vi "Configure.vi"(8 "error in (no error)":errorcluster, 11 "Insight in":refnum<class "Insight.lvclass">) -> (0 "error out":errorcluster, 3 "Insight out":refnum<class "Insight.lvclass">)   [LabVIEW 2014, in "Insight.lvclass"]
uses:
  Insight.lvclass
  Insight.lvclass/Insight.ctl
panel:
  out "Finished":bool
  out "Calibrating":bool
  in  "File Path Control":path=path "\\\\192.168.1.100\\data"
  in  "Aprox. Req. Sweep Rate (kHz)":dbl=50000.0
  in  "OK Button":bool
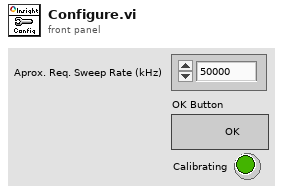
[diagram p1: front panel]
types:
  T1 = typedef "Telnet Session.ctl" = refnum<k1>
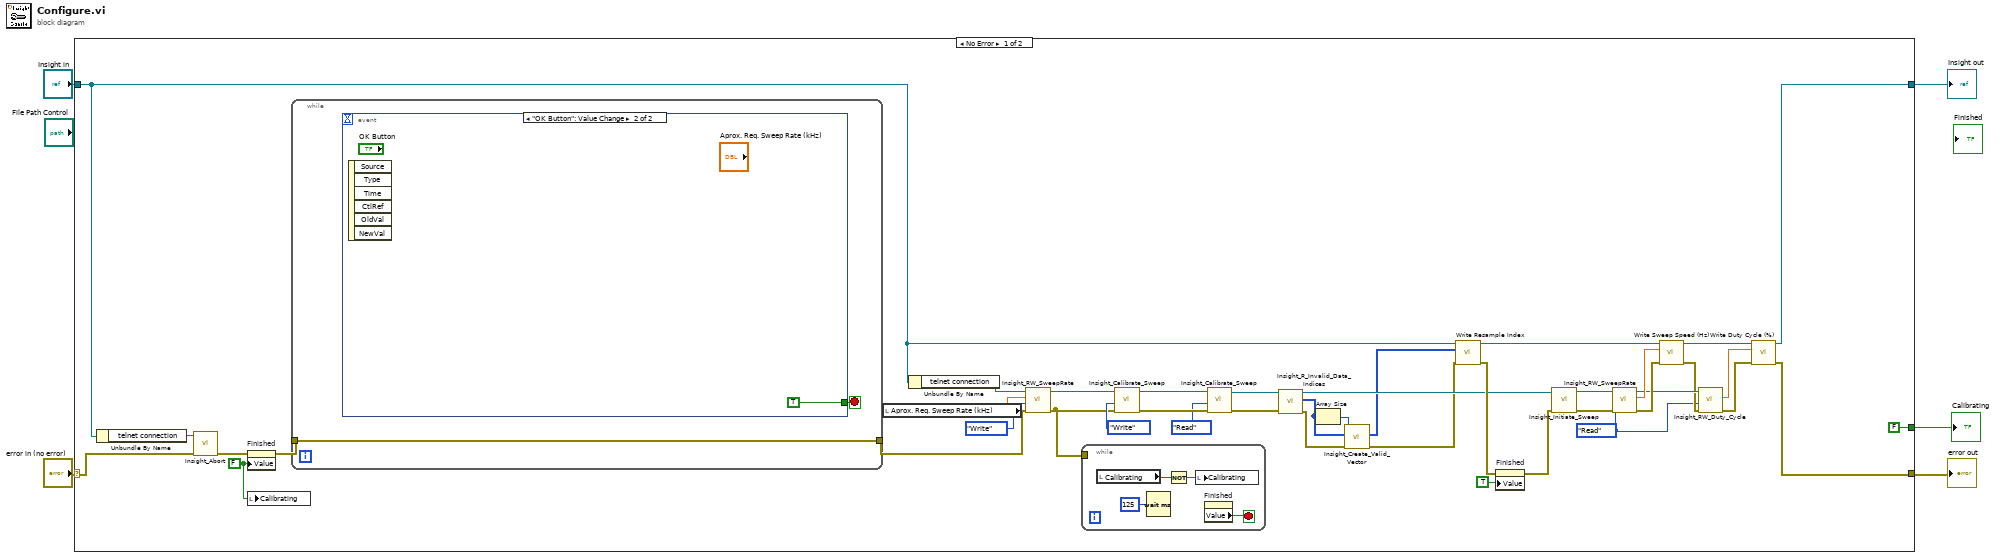
[diagram p0: block diagram]
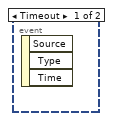
[diagram p2: hidden frame]
diagram:
  n1 = case shown="No Error" "error in (no error)" {
    selector: "error in (no error)" -> [w32 w56]
    tunnel: [w19 w56] -> w4
    tunnel: [w18 w55] -> w2
    tunnel: "Insight in" -> [w33 w55]
    tunnel: [FALSE _] -> w1
    frame No Error {
      w23 = enum8{"Write", "Read"}."Read" ("Mode (Read / Write)")
      w31 = FALSE ("Finished")
      n2 = Unbundle By Name(w33) -> ("telnet connection"=w34:T1)
      n3 = call "Insight_Abort.vi"("error in (no error)"=w32, "telnet connection"=w34) -> ("error out"=w35:errorcluster)  [unwired: 7 in, 2 out]
      n4 = property on="Finished" class="Bool (strict)"(error in=w35, "Value"=w31) -> (error out=w38:errorcluster)  [unwired: 1 in, 1 out]
      n5 = local write "Calibrating"(w31) -> ()
      n6 = while {
        tunnel: w38 -> [w52]
        tunnel: [w52] -> w41
        stop <- w53 stop-if-true
        n7 = event shown="[1] \"OK Button\": Value Change" {
          selector: _ -> [_ _]
          dyn-events: _ -> [_ _]
          timeout: _ -> [_ _]
          tunnel: [_ TRUE] -> w53
          event Timeout {
            n8 = event-data() -> ()  [unwired: 1 in, 3 out]
          }
          event "OK Button": Value Change {
            n9 = event-data() -> ()  [unwired: 1 in, 6 out]
          }
        }
      }
      n10 = local read "Aprox. Req. Sweep Rate (kHz)"() -> (w44:dbl)
      n11 = Unbundle By Name(w33) -> ("telnet connection"=w46:T1)
      n12 = call "Insight_RW_SweepRate.vi"("error in (no error)"=w41, "Mode (Read / Write)"=enum8{"Write", "Read"}."Write", "Sweep Rate (kHz)"=w44, "telnet connection"=w46) -> ("error out"=w40:errorcluster, "telnet  connection out"=w42:T1)  [unwired: 4 in, 2 out]
      n13 = while {
        tunnel: [w51] -> _
        tunnel: w40 -> [w51]
        stop <- w50 stop-if-true
        n14 = local read "Calibrating"() -> (w49:bool)
        n15 = Wait (ms)(milliseconds to wait=u32 125) -> ()  [unwired: 1 out]
        n16 = Not(x=w49) -> (.not. x?=w48:bool)
        n17 = local write "Calibrating"(w48) -> ()
        n18 = property on="Finished" class="Bool (strict)"() -> ("Value"=w50:bool)  [unwired: 2 in, 2 out]
      }
      n19 = call "Insight_Calibrate_Sweep.vi"("error in (no error)"=w40, "Mode (Read / Write)"=enum8{"Write", "Read"}."Write", "telnet connection"=w42) -> ("error out"=w16:errorcluster, "telnet  connection out"=w15:T1)  [unwired: 6 in, 1 out]
      n20 = call "Insight_Calibrate_Sweep.vi"("error in (no error)"=w16, "Mode (Read / Write)"=enum8{"Write", "Read"}."Read", "telnet connection"=w15) -> ("error out"=w10:errorcluster, "telnet  connection out"=w9:T1)  [unwired: 6 in, 1 out]
      n21 = call "Insight_R_Invalid_Data_Indices.vi"("error in (no error)"=w10, "telnet connection"=w9) -> ("error out"=w13:errorcluster, "Invalid Data Indices"=w11:i32[], "telnet  connection out"=w8:T1)  [unwired: 6 in, 1 out]
      n22 = Array Size(array=w11) -> (size(s)=w12:i32)
      n23 = call "Insight_Create_Valid_Vector.vi"("error in (no error)"=w13, "Invalid Data Indices"=w11, "total data length"=w12) -> ("error out"=w7:errorcluster, "Valid Vector"=w6:i32[])  [unwired: 7 in]
      n24 = call-dynamic "Write Resample Index.vi"("error in (no error)"=w7, "Resample Index"=w6, "Laser in"=w33) -> ("error out"=w37:errorcluster, "Laser out"=w26:refnum<class "Insight.lvclass">)  [unwired: 7 in]
      n25 = property on="Finished" class="Bool (strict)"(error in=w37, "Value"=TRUE ("Finished")) -> (error out=w36:errorcluster)  [unwired: 1 in, 1 out]
      n26 = call "Insight_Initiate_Sweep.vi"("error in (no error)"=w36, "telnet connection"=w8) -> ("error out"=w30:errorcluster, "telnet  connection out"=w29:T1)  [unwired: 7 in, 1 out]
      n27 = call "Insight_RW_SweepRate.vi"("error in (no error)"=w30, "Mode (Read / Write)"=w23, "telnet connection"=w29) -> ("error out"=w27:errorcluster, "Sweep Rate (kHz)"=w28:dbl, "telnet  connection out"=w25:T1)  [unwired: 5 in, 1 out]
      n28 = call-dynamic "Write Sweep Speed (Hz).vi"("error in (no error)"=w27, "Sweep Speed (Hz)"=w28, "Laser in"=w26) -> ("error out"=w24:errorcluster, "Laser out"=w20:refnum<class "Insight.lvclass">)  [unwired: 7 in]
      n29 = call "Insight_RW_Duty_Cycle.vi"("error in (no error)"=w24, "Mode (Read / Write)"=w23, "telnet connection"=w25) -> ("error out"=w22:errorcluster, "Duty Cycle(%)?"=w21:dbl)  [unwired: 5 in, 2 out]
      n30 = call-dynamic "Write Duty Cycle (%).vi"("error in (no error)"=w22, "Duty Cycle (%)"=w21, "Laser in"=w20) -> ("error out"=w19:errorcluster, "Laser out"=w18:refnum<class "Insight.lvclass">)  [unwired: 7 in]
    }
    frame Error {
    }
  }
  "error out" <- w4
  "Insight out" <- w2
  "Calibrating" <- w1
